vi "Priority String.vi"(11 "Execution:Priority":T1(ring)) -> (3 "Priority String":string)   [LabVIEW 2023, in "VIDoc Printer.lvlib" / "VIDoc Printer.lvclass"]
doc: "Converts the Execution Priority into a printable String."
uses:
  VIDoc Printer.lvclass
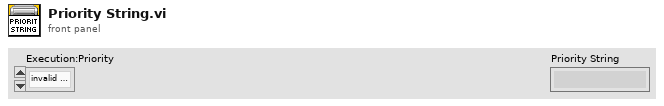
[diagram p1: front panel]
types:
  T1 = enum32{"invalid priority", "background priority", "normal priority", "above normal priority", "high priority", "time critical priority", "subroutine"}
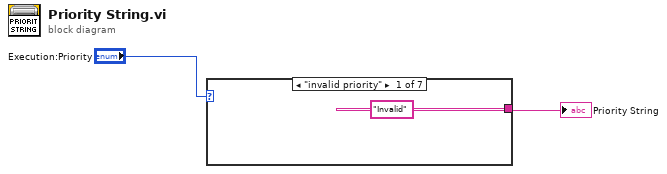
[diagram p0: block diagram]
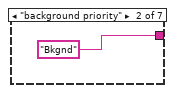
[diagram p2: hidden frame]
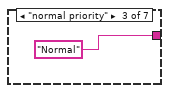
[diagram p3: hidden frame]
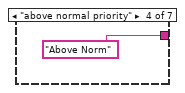
[diagram p4: hidden frame]
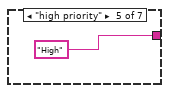
[diagram p5: hidden frame]
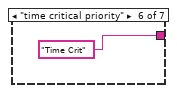
[diagram p6: hidden frame]
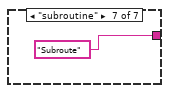
[diagram p7: hidden frame]
diagram:
  n1 = case shown="\"invalid priority\"" "Execution:Priority" {
    tunnel: ["Invalid" "Bkgnd" "Normal" "Above Norm" "High" "Time Crit" "Subroute"] -> w2
    frame "invalid priority" {
    }
    frame "background priority" {
    }
    frame "normal priority" {
    }
    frame "above normal priority" {
    }
    frame "high priority" {
    }
    frame "time critical priority" {
    }
    frame "subroutine" {
    }
  }
  "Priority String" <- w2
